vi "Dequeue SelfQueue Msg.vi"(8 "error in (no error)":errorcluster, 9 "Timeout":i32, 11 "ModuleAbstract in":refnum<class "ModuleAbstract.lvclass">) -> (0 "error out":errorcluster, 1 "Message Data":variant, 2 "Message":string, 3 "ModuleAbstract out":refnum<class "ModuleAbstract.lvclass">)   [LabVIEW 2019, in "ModuleAbstract.lvlib" / "ModuleAbstract.lvclass"]
uses:
  ModuleAbstract.lvclass
  ModuleAbstract.lvclass/ModuleAbstract.ctl
  Utilities/LV_Lib/Message Queue/Message Queue.lvlib
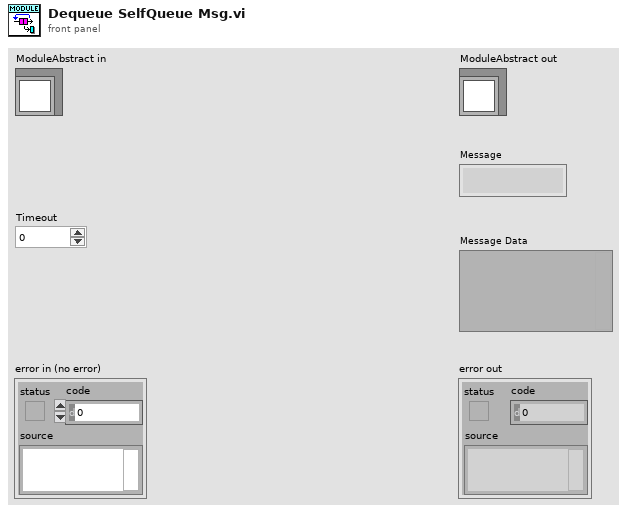
[diagram p1: front panel]
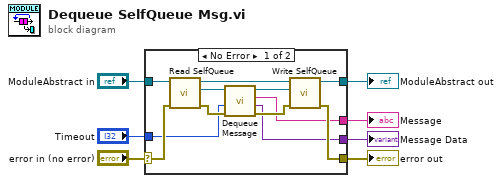
[diagram p0: block diagram]
diagram:
  n1 = case shown="No Error" "error in (no error)" {
    selector: "error in (no error)" -> [w12 w21]
    tunnel: [w11 w21] -> w6
    tunnel: [w13 w20] -> w4
    tunnel: "ModuleAbstract in" -> [w14 w20]
    tunnel: [w10 _] -> w3
    tunnel: [w9 _] -> w2
    tunnel: "Timeout" -> [w8 _]
    frame No Error {
      n2 = call "Read SelfQueue.vi"("error in (no error)"=w12, "ModuleAbstract in"=w14) -> ("error out"=w16:errorcluster, "SelfQueue"=w19:refnum<queue>, "ModuleAbstract out"=w17:refnum<class "ModuleAbstract.lvclass">)  [unwired: 7 in]
      n3 = call "Dequeue Message.vi"("error in (no error)"=w16, "timeout in ms (-1)"=w8, "Message Queue"=w19) -> ("error out"=w15:errorcluster, "Message Data"=w9:variant, "Message"=w10:string, "dup Message Queue"=w18:refnum<queue>)  [unwired: 5 in]
      n4 = call "Write SelfQueue.vi"("error in (no error)"=w15, "SelfQueue"=w18, "ModuleAbstract in"=w17) -> ("error out"=w11:errorcluster, "ModuleAbstract out"=w13:refnum<class "ModuleAbstract.lvclass">)  [unwired: 7 in]
    }
    frame Error {
    }
  }
  "error out" <- w6
  "ModuleAbstract out" <- w4
  "Message" <- w3
  "Message Data" <- w2
